vi "Memory.Pointer.Error Handling.Get Error Info.vi"(11 "error":T1) -> (2 "description":string, 3 "code":i32)   [LabVIEW 2016, in "LabVIEW Memory Manager.lvlib" / "Memory.Pointer.Void.lvclass"]
uses:
  Memory.Pointer.Void.lvclass
  Typedefs/Memory.Pointer.Error Codes.ctl
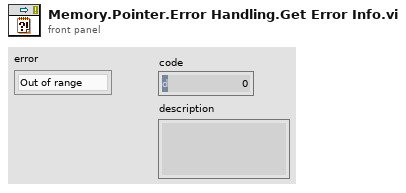
[diagram p1: front panel]
types:
  T1 = typedef "LabVIEW Memory Manager.lvlib/Memory.Pointer.Void.lvclass/Memory.Pointer.Error Codes.ctl" = enum16{"Out of range"}
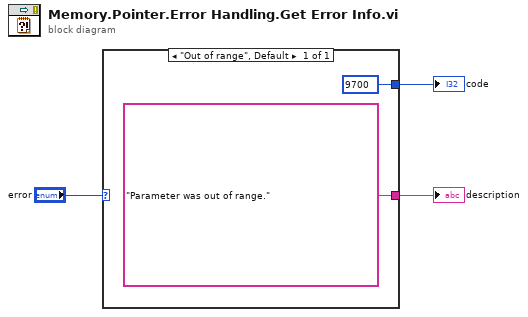
[diagram p0: block diagram]
diagram:
  n1 = case shown="\"Out of range\", Default" "error" {
    tunnel: ["Parameter was out of range."] -> w2
    tunnel: [9700 ("code")] -> w1
    frame "Out of range", Default {
    }
  }
  "description" <- w2
  "code" <- w1
